vi "ADB-Serial_WrRd_orig.vi"(5 "ReadInterval(mSec)":u32=75, 7 "Timeout(Sec)":dbl=5.0, 8 "error in (no error)":errorcluster, 9 "PassString":string="PASS", 10 "Command":string, 11 "ComPort":refnum<visa-resource-name>="COM10") -> (0 "error out":errorcluster, 2 "PASS":bool, 3 "received":string)   [LabVIEW 2018]
uses:
  <vilib>/Instr/_visa.llb/VISA Configure Serial Port (Instr).vi
panel:
  out "concatenated string":string
  # "ADB Serial W/R"
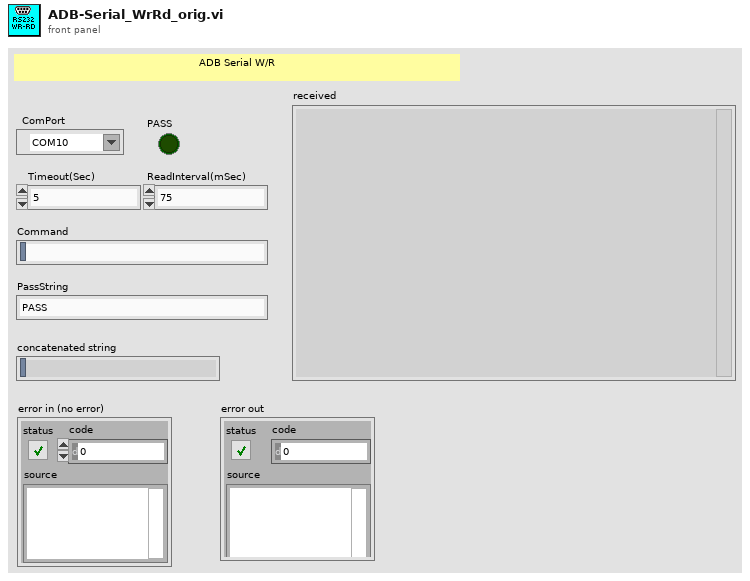
[diagram p1: front panel]
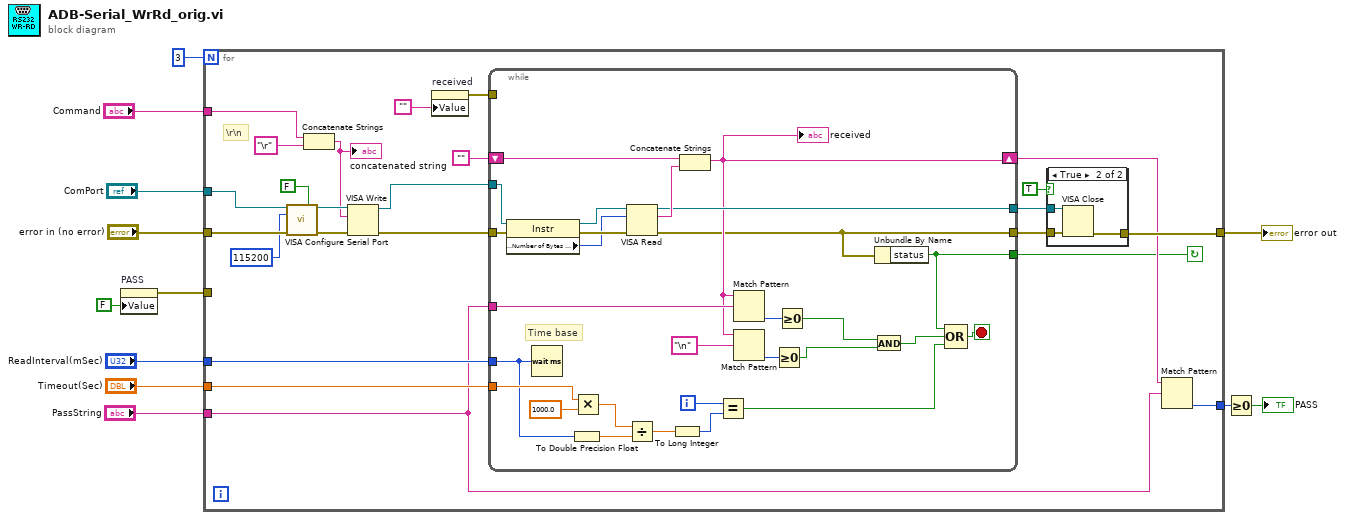
[diagram p0: block diagram]
diagram:
  n1 = property on="PASS" class="Bool (strict)"("Value"=FALSE ("PASS")) -> (error out=w2:errorcluster)  [unwired: 2 in, 1 out]
  n2 = for {
    N: 3 -> [_]
    tunnel: "ComPort" -> [w36]
    tunnel: "ReadInterval(mSec)" -> [w35]
    tunnel: [w34] -> w9
    tunnel: "Timeout(Sec)" -> [w29]
    tunnel: "PassString" -> [w23]
    tunnel: "Command" -> [w18]
    tunnel: "error in (no error)" -> [w33]
    tunnel: [w28] -> w3
    tunnel: w2 -> [_]
    stop <- w14 continue-if-true
    # "\\r\\n"
    n3 = call-poly "VISA Configure Serial Port"("VISA resource name"=w36, "Enable Termination\nChar (T)"=FALSE ("Enable Termination\nChar (T)"), "baud rate (9600)"=u32 115200 ("Serial Settings:Baud Rate"), "error in (no error)"=w33) -> ("VISA resource name out"=w31:refnum<visa-resource-name>, "error out"=w30:errorcluster)  [unwired: 10 in]
    n4 = Concatenate Strings(w18, "\r" ("string")) -> (w19:string)
    "concatenated string" <- w19
    n5 = VISA Write(VISA resource name=w31, write buffer=w19, error in (no error)=w30) -> (VISA resource name out=w24:refnum<visa-resource-name>, error out=w15:errorcluster)  [unwired: 1 out]
    n6 = property on="received" class="Str"("Value"="") -> (error out=w16:errorcluster)  [unwired: 2 in, 1 out]
    n7 = while {
      tunnel: w15 -> [w68]
      tunnel: w24 -> [w67]
      tunnel: [w42] -> w26
      shift-right: [w46] -> w20
      shift-left: "" -> [w64]
      tunnel: [w62] -> w27
      tunnel: w35 -> [w55]
      tunnel: w29 -> [w58]
      tunnel: w23 -> [w49]
      tunnel: [w41] -> w14
      tunnel: w16 -> [_]
      i -> [w59]
      stop <- w61 stop-if-true
      # "Time base"
      n8 = property class="Instr"(reference=w67, error in=w68) -> (reference out=w65:refnum<visa-resource-name>, error out=w66:errorcluster, "Serial Settings:Number of Bytes at Serial Port"=w51:u32)
      n9 = Wait (ms)(milliseconds to wait=w55) -> ()  [unwired: 1 out]
      n10 = To Double Precision Float(number=w55) -> (double precision float=w52:dbl)
      n11 = Multiply(x=w58, y=1000.0) -> (x*y=w56:dbl)
      n12 = VISA Read(VISA resource name=w65, byte count=w51, error in (no error)=w66) -> (VISA resource name out=w62:refnum<visa-resource-name>, read buffer=w63:string, error out=w42:errorcluster)  [unwired: 1 out]
      n13 = Divide(x=w56, y=w52) -> (x/y=w54:dbl)
      n14 = To Long Integer(number=w54) -> (32bit integer=w53:i32)
      n15 = Concatenate Strings(w64, w63) -> (w46:string)
      "received" <- w46
      n16 = Equal?(x=w59, y=w53) -> (x = y?=w60:bool)
      n17 = Match Pattern(string=w46, regular expression=w49) -> (offset past match=w50:i32)  [unwired: 1 in, 3 out]
      n18 = Match Pattern(string=w46, regular expression="\n") -> (offset past match=w48:i32)  [unwired: 1 in, 3 out]
      n19 = Greater Or Equal To 0?(x=w48) -> (x >= 0?=w43:bool)
      n20 = Greater Or Equal To 0?(x=w50) -> (x >= 0?=w44:bool)
      n21 = And(x=w44, y=w43) -> (x .and. y?=w47:bool)
      n22 = Unbundle By Name(w42) -> ("status"=w41:bool)
      n23 = Compound Arithmetic op=OR(w41, w47, w60) -> (w61:bool)
    }
    n24 = case shown="True" TRUE {
      tunnel: [w37 w40] -> w28
      tunnel: w27 -> [_ w39]
      tunnel: w26 -> [w37 w38]
      frame False {
      }
      frame True {
        n25 = VISA Close(VISA resource name=w39, error in (no error)=w38) -> (error out=w40:errorcluster)
      }
    }
    n26 = Match Pattern(string=w20, regular expression=w23) -> (offset past match=w34:i32)  [unwired: 1 in, 3 out]
  }
  "error out" <- w3
  n27 = Greater Or Equal To 0?(x=w9) -> (x >= 0?=→"PASS":bool)
